vi "ICNC Get Buffer Status.vi"(8 "error in (no error)":errorcluster caption="entrée d'erreur (pas d'erreur)", 11 "FreeBufferSpace":u32) -> (0 "error out":errorcluster caption="sortie d'erreur", 2 "function return":u32, 3 "FreeBufferSpace out":u32)   [LabVIEW 2012, in "ICNC2.lvlib"]
doc: "DWORD ICNC_GetBufferStatus( DWORD *FreeBufferSpace);"
uses:
  <userlib>/ICNC/ICNC2.lvlib
  <userlib>/ICNC/ICNC2.dll
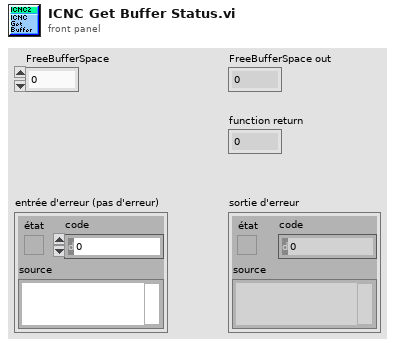
[diagram p1: front panel]
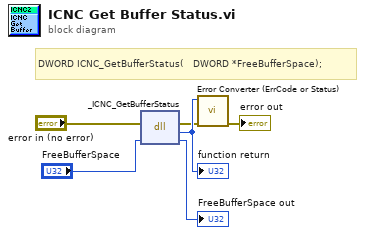
[diagram p0: block diagram]
diagram:
  # "DWORD ICNC_GetBufferStatus(   DWORD *FreeBufferSpace);"
  n1 = dll-call lib="C:/Program Files (x86)/National Instruments/LabVIEW 2012/user.lib/ICNC/ICNC2.*" fn="_ICNC_GetBufferStatus"(error in="error in (no error)", "FreeBufferSpace"="FreeBufferSpace") -> (error out=w2:errorcluster, w6:u32, "FreeBufferSpace"=→"FreeBufferSpace out":u32)  [unwired: 2 in, 1 out]
  "function return" <- w6
  n2 = call <userlib>:"Error Converter (ErrCode or Status).vi"("error in (no error)"=w2, "error code"=w6) -> ("error out"=→"error out":errorcluster)  [unwired: 9 in]
